vi "PusherControlLoop.vi"   [LabVIEW 2014, in "PusherLib.lvlib"]
uses:
  PusherLib.lvlib
  PusherRefs.ctl
types:
  T1 = typedef "PusherLib.lvlib/PusherRefs.ctl" = enum16{"PusherLeft", "PusherRight", "PusherStringPot"}
  T2 = typedef "WPI_MotorControlDeviceRef.ctl" = cluster{"DeviceStatus":errorcluster, "Type":T3, "PWM":cluster{"Controller":T4, "PWM Channel":T5, "DeadBand":T6}, "CAN":cluster{"Device Number":u8, "Control Mode":T7, "Semaphore":T8, "Max Vout":dbl, "TalonSRX Control Mode":T9}, "Invert":bool, "TransformRef":T10, "InvTransformRef":T10}
  T3 = typedef "WPI_MotorControlType.ctl" = enum16{"PWM", "CAN", "CANTalonSRX"}
  T4 = typedef "FPGA_TypedefDigitalModule.ctl" = enum16{"Controller 1"}
  T5 = typedef "FPGA_DIOPWMChannel.ctl" = enum8{"PWM 0", "PWM 1", "PWM 2", "PWM 3", "PWM 4", "PWM 5", "PWM 6", "PWM 7", "PWM 8", "PWM 9", "PWM MXP 0", "PWM MXP 1", "PWM MXP 2", "PWM MXP 3", "PWM MXP 4", "PWM MXP 5", "PWM MXP 6", "PWM MXP 7", "PWM MXP 8", "PWM MXP 9", "Invalid"}
  T6 = typedef "WPI_PWMDeadband.ctl" = cluster{"Name":string, "maxPositivePwm":i32, "minPositivePwm":i32, "centerPwm":i32, "maxNegativePwm":i32, "minNegativePwm":i32, "angularRange":u16}
  T7 = typedef "WPI_CANJaguar_ControlMode.ctl" = enum8{"Percent VBus", "Current", "Speed", "Position", "Voltage"}
  T8 = typedef "Semaphore RefNum" = refnum<k1>
  T9 = typedef "WPI_CANTalonSRX_APIControlMode.ctl" = enum8{"Percent VBus", "Speed", "Position", "Slave", "Unchanged / Invalid"}
  T10 = typedef "WPI_PWMTransform_ConPane.ctl" = refnum<vi>
  T11 = typedef "WPI_PotentiometerDevRef.ctl" = cluster{"DevStatus":errorcluster, "Controller":T12, "Analog Channel":T13, "Invert Output":bool}
  T12 = typedef "FPGA_TypedefAnalogModule.ctl" = enum16{"Controller 1"}
  T13 = typedef "FPGA_AIChannel.ctl" = enum8{"AI 0", "AI 1", "AI 2", "AI 3", "AI MXP 0", "AI MXP 1", "AI MXP 2", "AI MXP 3", "Invalid"}
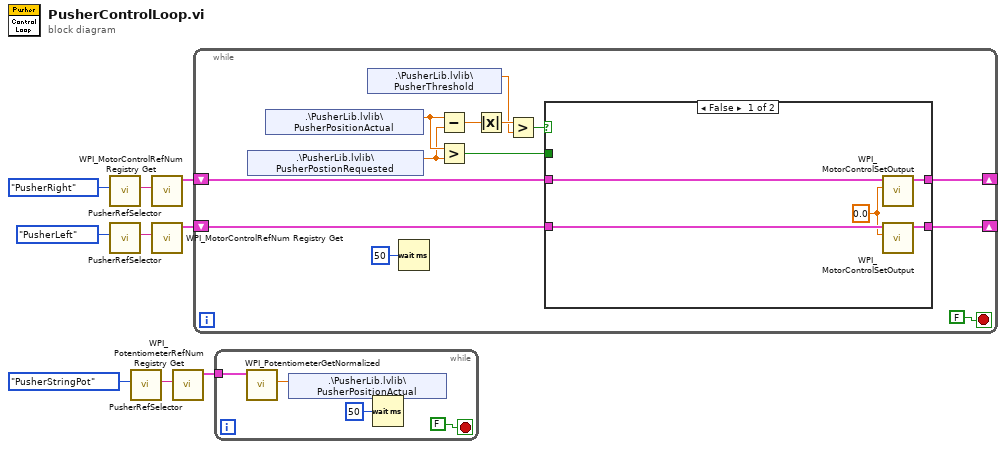
[diagram p0: block diagram]
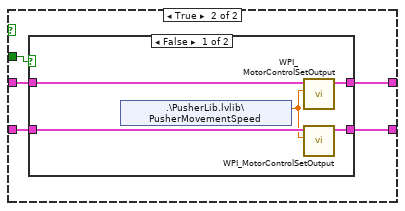
[diagram p2: hidden frame]
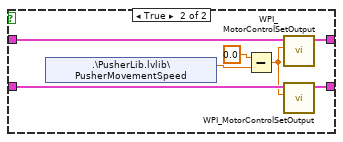
[diagram p3: hidden frame]
diagram:
  n1 = call "PusherRefSelector.vi"("PusherRefs"=PusherRefs."PusherRight") -> ("Refnum"=w6:string)  [unwired: 10 in]
  n2 = call "PusherRefSelector.vi"("PusherRefs"=PusherRefs."PusherLeft") -> ("Refnum"=w9:string)  [unwired: 10 in]
  n3 = call "PusherRefSelector.vi"("PusherRefs"=PusherRefs."PusherStringPot") -> ("Refnum"=w2:string)  [unwired: 10 in]
  n4 = call <vilib>:"WPI_MotorControlRefNum Registry Get.vi"("refnum name"=w6) -> ("MotorControlDevRef"=w4:T2)  [unwired: 9 in, 1 out]
  n5 = call <vilib>:"WPI_MotorControlRefNum Registry Get.vi"("refnum name"=w9) -> ("MotorControlDevRef"=w5:T2)  [unwired: 9 in, 1 out]
  n6 = call <vilib>:"WPI_PotentiometerRefNum Registry Get.vi"("refnum name"=w2) -> ("PotDevRef"=w1:T11)  [unwired: 9 in, 1 out]
  n7 = while {
    shift-right: [w14] -> _
    shift-left: w5 -> [w15]
    shift-right: [w12] -> _
    shift-left: w4 -> [w13]
    stop <- FALSE stop-if-true
    n8 = shared-variable ".\\PusherLib.lvlib\\PusherPostionRequested"() -> (w17:dbl)  [unwired: 1 in, 1 out]
    n9 = shared-variable ".\\PusherLib.lvlib\\PusherPositionActual"() -> (w18:dbl)  [unwired: 1 in, 1 out]
    n10 = shared-variable ".\\PusherLib.lvlib\\PusherThreshold"() -> (w20:dbl)  [unwired: 1 in, 1 out]
    n11 = Wait (ms)(milliseconds to wait=u32 50) -> ()  [unwired: 1 out]
    n12 = Subtract(x=w18, y=w17) -> (x-y=w22:dbl)
    n13 = Greater?(x=w18, y=w17) -> (0:w16:bool)
    n14 = Absolute Value(x=w22) -> (abs(x)=w21:dbl)
    n15 = Greater?(x=w21, y=w20) -> (0:w19:bool)
    n16 = case shown="False" w19 {
      tunnel: w16 -> [_ w32]
      tunnel: w15 -> [w25 w31]
      tunnel: [w24 w30] -> w14
      tunnel: [w26 w29] -> w12
      tunnel: w13 -> [w27 w28]
      frame False {
        w23 = 0.0 ("Output")
        n17 = call <vilib>:"WPI_MotorControlSetOutput.vi"("Output"=w23, "MotorControlDevRef"=w27) -> ("MotorControlDevRef"=w26:T2)  [unwired: 7 in, 2 out]
        n18 = call <vilib>:"WPI_MotorControlSetOutput.vi"("Output"=w23, "MotorControlDevRef"=w25) -> ("MotorControlDevRef"=w24:T2)  [unwired: 7 in, 2 out]
      }
      frame True {
        n19 = case shown="False" w32 {
          tunnel: w31 -> [w36 w44]
          tunnel: [w34 w43] -> w30
          tunnel: [w35 w41] -> w29
          tunnel: w28 -> [w37 w42]
          frame False {
            n20 = shared-variable ".\\PusherLib.lvlib\\PusherMovementSpeed"() -> (w33:dbl)  [unwired: 1 in, 1 out]
            n21 = call <vilib>:"WPI_MotorControlSetOutput.vi"("Output"=w33, "MotorControlDevRef"=w37) -> ("MotorControlDevRef"=w35:T2)  [unwired: 7 in, 2 out]
            n22 = call <vilib>:"WPI_MotorControlSetOutput.vi"("Output"=w33, "MotorControlDevRef"=w36) -> ("MotorControlDevRef"=w34:T2)  [unwired: 7 in, 2 out]
          }
          frame True {
            n23 = shared-variable ".\\PusherLib.lvlib\\PusherMovementSpeed"() -> (w39:dbl)  [unwired: 1 in, 1 out]
            n24 = Subtract(x=0.0, y=w39) -> (x-y=w38:dbl)
            n25 = call <vilib>:"WPI_MotorControlSetOutput.vi"("Output"=w38, "MotorControlDevRef"=w42) -> ("MotorControlDevRef"=w41:T2)  [unwired: 7 in, 2 out]
            n26 = call <vilib>:"WPI_MotorControlSetOutput.vi"("Output"=w38, "MotorControlDevRef"=w44) -> ("MotorControlDevRef"=w43:T2)  [unwired: 7 in, 2 out]
          }
        }
      }
    }
  }
  n27 = while {
    tunnel: w1 -> [w47]
    stop <- FALSE stop-if-true
    n28 = call <vilib>:"WPI_PotentiometerGetNormalized.vi"("PotDevRef"=w47) -> ("Normalized Value"=w46:dbl)  [unwired: 8 in, 2 out]
    n29 = shared-variable ".\\PusherLib.lvlib\\PusherPositionActual"(w46) -> ()  [unwired: 1 in, 1 out]
    n30 = Wait (ms)(milliseconds to wait=u32 50) -> ()  [unwired: 1 out]
  }
